vi "configuration_write.vi"(8 "error in (no error)":errorcluster, 10 "configuration":variant, 11 "lv-build in":refnum<class "lv-builder-default.lvclass">) -> (0 "error out":errorcluster, 3 "lv-build out":refnum<class "lv-builder-default.lvclass">)   [LabVIEW 2015, in "lv-builder-default.lvclass"]
uses:
  lv-builder-default.lvclass
  lv-builder-default.lvclass/lv-builder-default.ctl
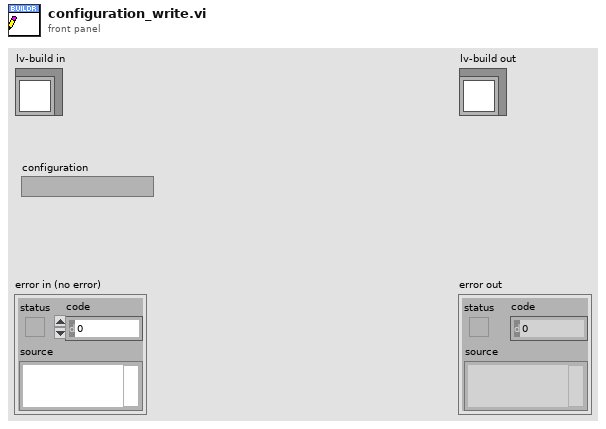
[diagram p1: front panel]
types:
  T1 = typedef "lv-builder-default.lvlib/configuration.ctl" = cluster{"project_file":string, "lvlibp_directory":string, "zip_directory":string, "lvlib_directory":string, "update_version_vi":string, "installer_post_file":string, "distribution_folder":string, "dependencies_folder":string, "version":string, "bin_folder":string, "lvlib_post_action":u16, "installer_post_action":u16, "application_post_action":u16, "zip_post_action":u16}
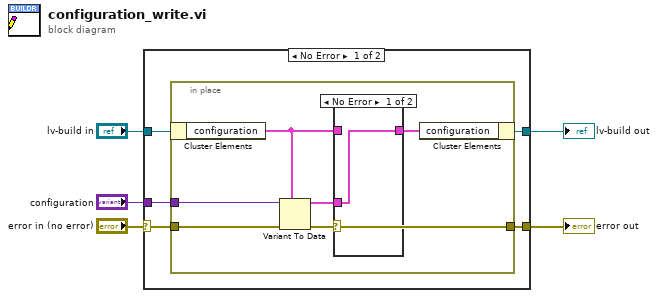
[diagram p0: block diagram]
diagram:
  n1 = case shown="No Error" "error in (no error)" {
    selector: "error in (no error)" -> [w9 w20]
    tunnel: "lv-build in" -> [w8 w19]
    tunnel: [w7 w19] -> w4
    tunnel: "configuration" -> [w10 _]
    tunnel: [w6 w20] -> w2
    frame No Error {
      n2 = in-place {
        in-place-border: w10 -> [w16]
        in-place-border: w9 -> [w15]
        in-place-border: [w12] -> w6
        n3 = in-place-cluster #1(w8) -> ("configuration"=w11:T1)
        n4 = Variant To Data(error in=w15, type=w11, Variant=w16) -> (data=w14:T1, error out=w12:errorcluster)
        n5 = case shown="No Error" w12 {
          tunnel: w14 -> [w17 _]
          tunnel: w11 -> [_ w18]
          tunnel: [w17 w18] -> w13
          frame No Error {
          }
          frame Error {
          }
        }
        n6 = in-place-cluster #1("configuration"=w13) -> (w7:refnum<class "lv-builder-default.lvclass">)
      }
    }
    frame Error {
    }
  }
  "error out" <- w2
  "lv-build out" <- w4
